vi "Prueba GAP.vi"(11 "Class 2.lvclass":refnum<class "Class 2.lvclass">) -> (3 "Class 2.lvclass 2":refnum<class "Class 2.lvclass">)   [LabVIEW 2019, in "Class 2.lvclass"]
uses:
  Class 2.lvclass
  Class 2.lvclass/Class 2.ctl
panel:
  in  "stop":bool
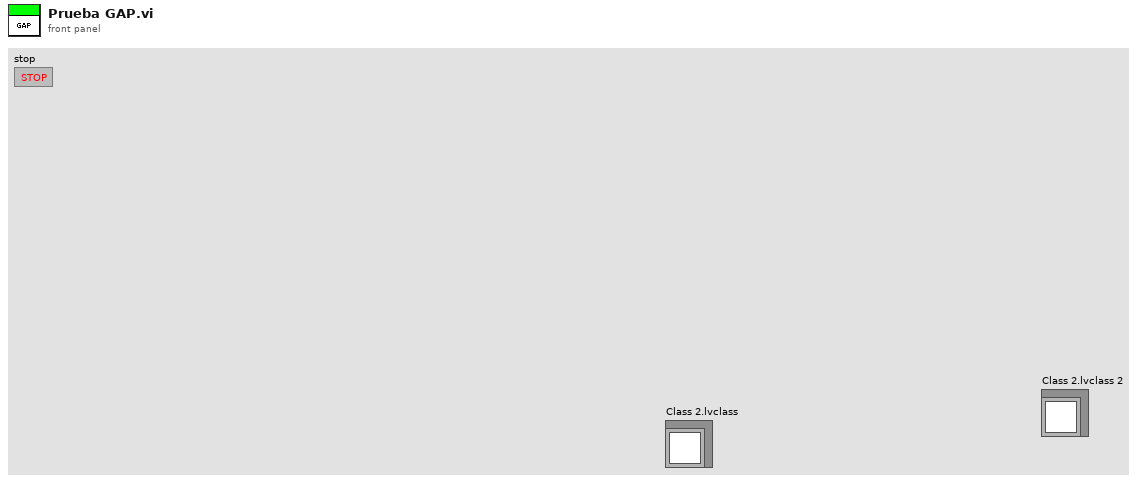
[diagram p1: front panel]
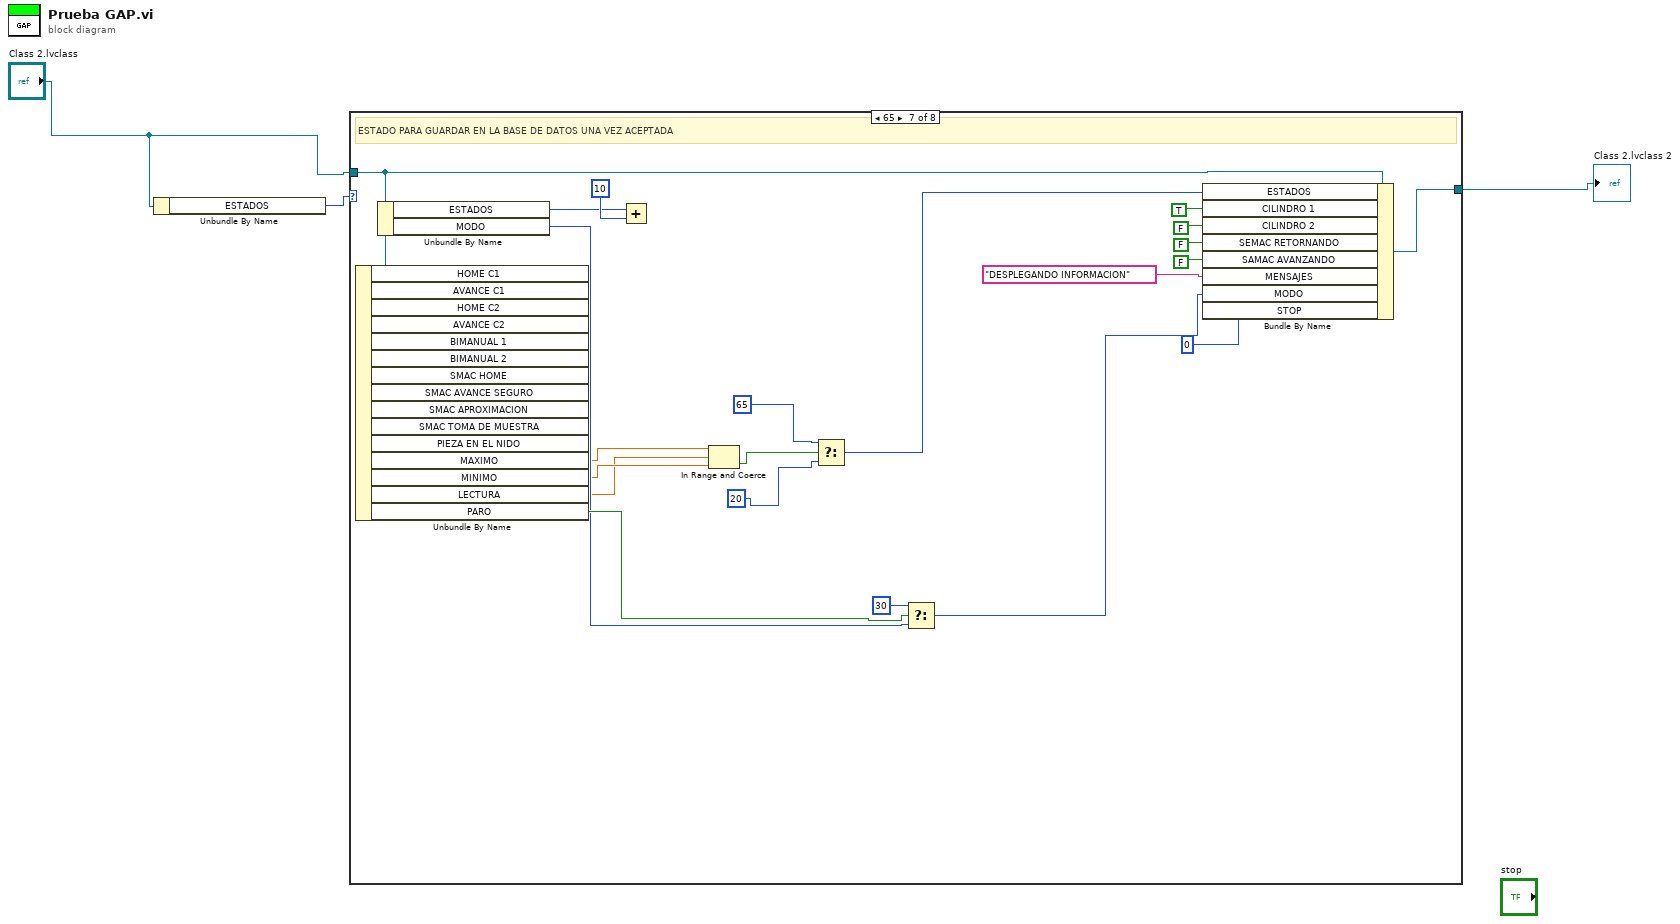
[diagram p0: block diagram]
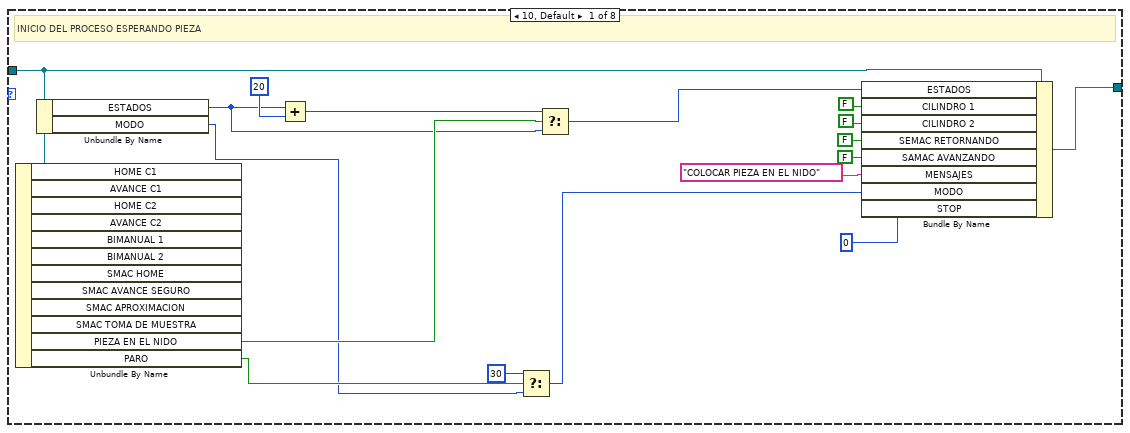
[diagram p2: hidden frame]
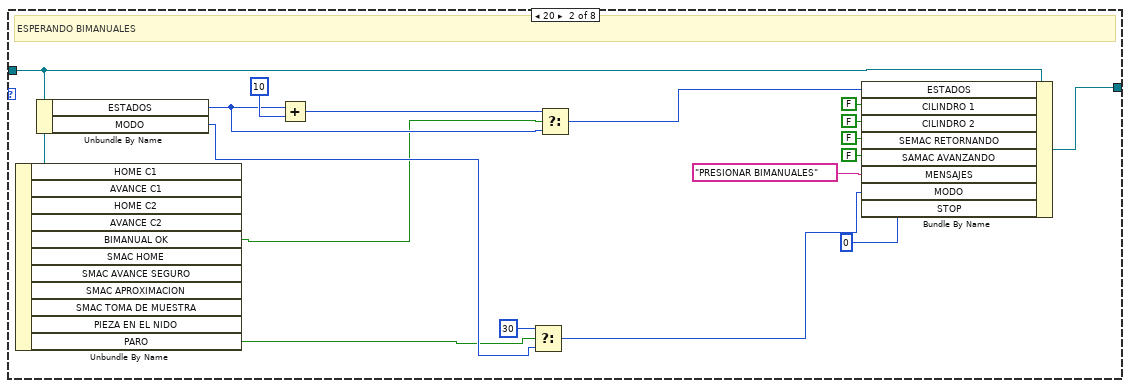
[diagram p3: hidden frame]
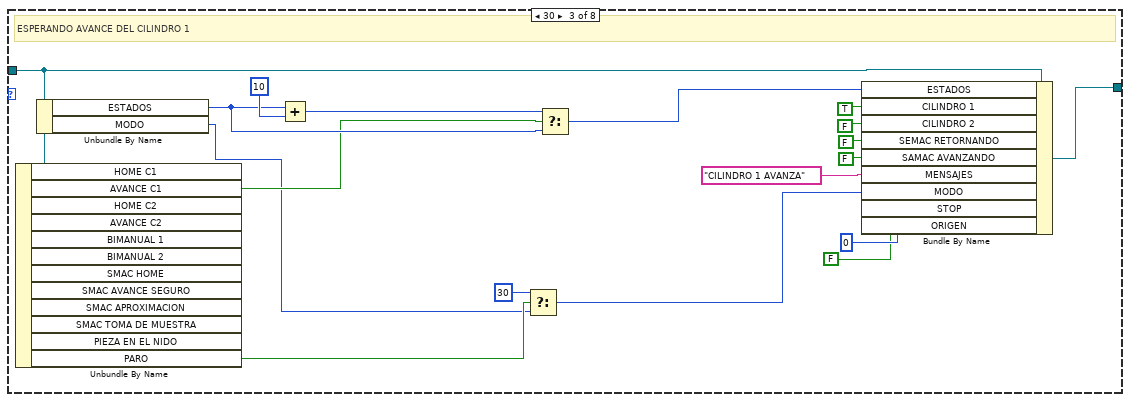
[diagram p4: hidden frame]
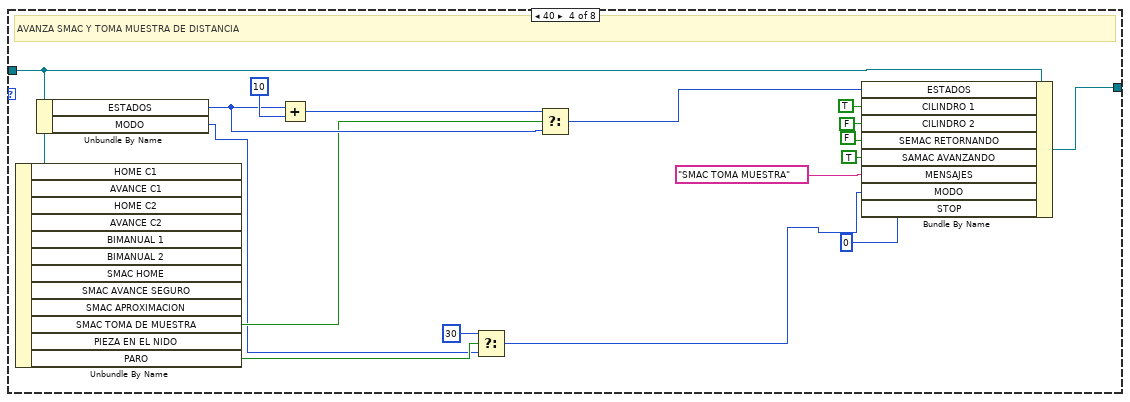
[diagram p5: hidden frame]
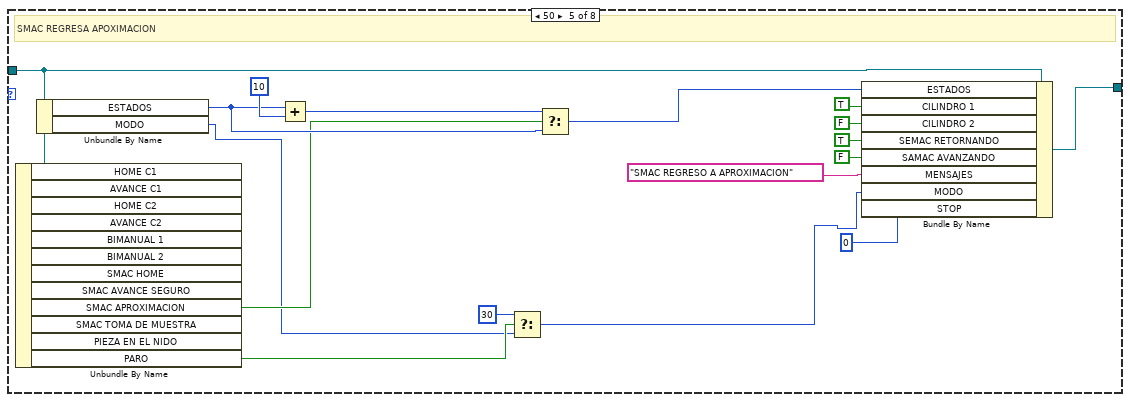
[diagram p6: hidden frame]
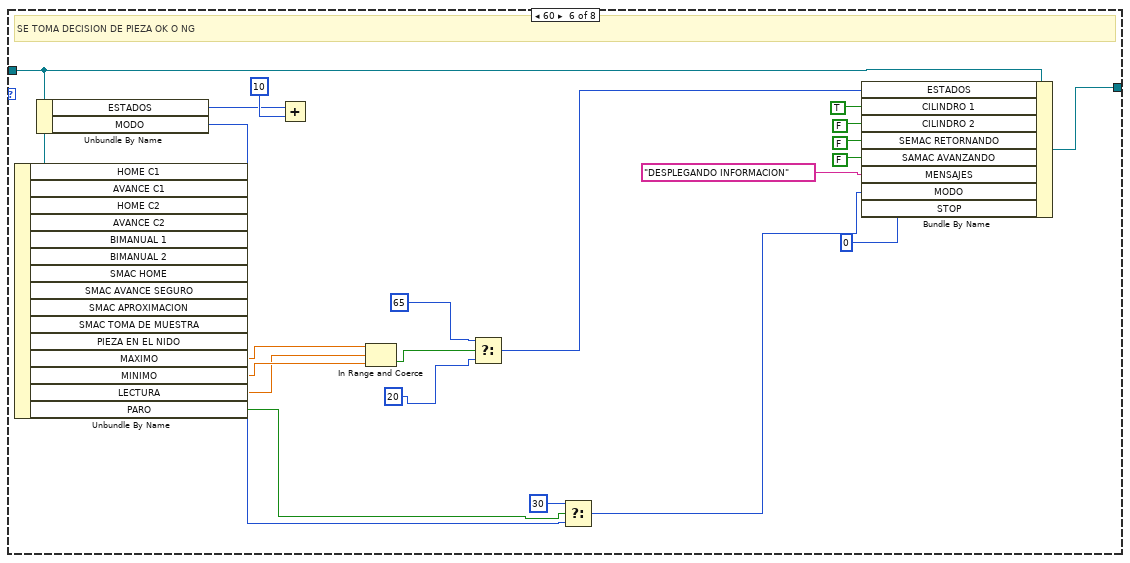
[diagram p7: hidden frame]
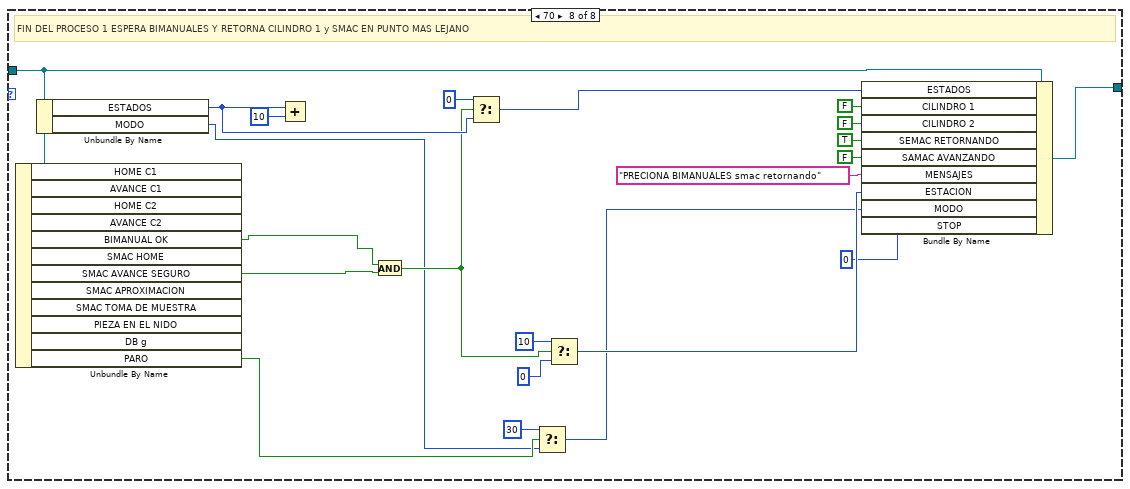
[diagram p8: hidden frame]
diagram:
  n1 = Unbundle By Name("Class 2.lvclass") -> ("ESTADOS"=w3:i16)
  n2 = case shown="65" w3 {
    tunnel: "Class 2.lvclass" -> [w16 w32 w50 w67 w84 w108 w129 w151]
    tunnel: [w20 w37 w55 w72 w89 w110 w131 w153] -> w1
    frame 10, Default {
      # "INICIO DEL PROCESO ESPERANDO PIEZA"
      n3 = Unbundle By Name(w16) -> ("PIEZA EN EL NIDO"=w14:bool, "PARO"=w9:bool)  [unwired: 10 out]
      n4 = Unbundle By Name(w16) -> ("ESTADOS"=w8:i16, "MODO"=w6:i16)
      n5 = Add(x=w8, y=i16 20) -> (x+y=w18:i16)
      n6 = Select(t=i16 30, s=w9, f=w6) -> (s? t:f=w4:i16)
      n7 = Select(t=w18, s=w14, f=w8) -> (s? t:f=w17:i16)
      n8 = Bundle By Name(cluster=w16, "ESTADOS"=w17, "CILINDRO 1"=FALSE ("SALIDAS.CILINDRO 1"), "CILINDRO 2"=FALSE ("SALIDAS.CILINDRO 2"), "SEMAC RETORNANDO"=FALSE ("SALIDAS.SEMAC RETORNANDO"), "SAMAC AVANZANDO"=FALSE ("SALIDAS.SAMAC AVANZANDO"), "MENSAJES"="COLOCAR PIEZA EN EL NIDO" ("SALIDAS.MENSAJES"), "MODO"=w4, "STOP"=i16 0 ("MAQ DE ESTADOS.MODO")) -> (w20:refnum<class "Class 2.lvclass">)
    }
    frame 20 {
      # "ESPERANDO BIMANUALES"
      n9 = Unbundle By Name(w32) -> ("BIMANUAL OK"=w21:bool, "PARO"=w24:bool)  [unwired: 9 out]
      n10 = Unbundle By Name(w32) -> ("ESTADOS"=w34:i16, "MODO"=w25:i16)
      n11 = Add(x=w34, y=i16 10) -> (x+y=w35:i16)
      n12 = Select(t=i16 30, s=w24, f=w25) -> (s? t:f=w23:i16)
      n13 = Select(t=w35, s=w21, f=w34) -> (s? t:f=w33:i16)
      n14 = Bundle By Name(cluster=w32, "ESTADOS"=w33, "CILINDRO 1"=FALSE ("SALIDAS.CILINDRO 1"), "CILINDRO 2"=FALSE ("SALIDAS.CILINDRO 2"), "SEMAC RETORNANDO"=FALSE ("SALIDAS.SEMAC RETORNANDO"), "SAMAC AVANZANDO"=FALSE ("SALIDAS.SAMAC AVANZANDO"), "MENSAJES"="PRESIONAR BIMANUALES" ("SALIDAS.MENSAJES"), "MODO"=w23, "STOP"=i16 0 ("MAQ DE ESTADOS.STOP")) -> (w37:refnum<class "Class 2.lvclass">)
    }
    frame 30 {
      # "ESPERANDO AVANCE DEL CILINDRO 1"
      n15 = Unbundle By Name(w50) -> ("AVANCE C1"=w44:bool, "PARO"=w41:bool)  [unwired: 10 out]
      n16 = Unbundle By Name(w50) -> ("ESTADOS"=w52:i16, "MODO"=w40:i16)
      n17 = Add(x=w52, y=i16 10) -> (x+y=w53:i16)
      n18 = Select(t=i16 30, s=w41, f=w40) -> (s? t:f=w42:i16)
      n19 = Select(t=w53, s=w44, f=w52) -> (s? t:f=w51:i16)
      n20 = Bundle By Name(cluster=w50, "ESTADOS"=w51, "CILINDRO 1"=TRUE ("SALIDAS.CILINDRO 1"), "CILINDRO 2"=FALSE ("SALIDAS.CILINDRO 2"), "SEMAC RETORNANDO"=FALSE ("SALIDAS.SEMAC RETORNANDO"), "SAMAC AVANZANDO"=FALSE ("SALIDAS.SAMAC AVANZANDO"), "MENSAJES"="CILINDRO 1 AVANZA" ("SALIDAS.MENSAJES"), "MODO"=w42, "STOP"=i16 0 ("MAQ DE ESTADOS.STOP"), "ORIGEN"=FALSE ("PROCESO.ORIGEN")) -> (w55:refnum<class "Class 2.lvclass">)
    }
    frame 40 {
      # "AVANZA SMAC Y TOMA MUESTRA DE DISTANCIA"
      n21 = Unbundle By Name(w67) -> ("SMAC TOMA DE MUESTRA"=w61:bool, "PARO"=w59:bool)  [unwired: 10 out]
      n22 = Unbundle By Name(w67) -> ("ESTADOS"=w69:i16, "MODO"=w58:i16)
      n23 = Add(x=w69, y=i16 10) -> (x+y=w70:i16)
      n24 = Select(t=i16 30, s=w59, f=w58) -> (s? t:f=w57:i16)
      n25 = Select(t=w70, s=w61, f=w69) -> (s? t:f=w68:i16)
      n26 = Bundle By Name(cluster=w67, "ESTADOS"=w68, "CILINDRO 1"=TRUE ("SALIDAS.CILINDRO 1"), "CILINDRO 2"=FALSE ("SALIDAS.CILINDRO 2"), "SEMAC RETORNANDO"=FALSE ("SALIDAS.SEMAC RETORNANDO"), "SAMAC AVANZANDO"=TRUE ("SALIDAS.SAMAC AVANZANDO"), "MENSAJES"="SMAC TOMA MUESTRA" ("SALIDAS.MENSAJES"), "MODO"=w57, "STOP"=i16 0 ("MAQ DE ESTADOS.STOP")) -> (w72:refnum<class "Class 2.lvclass">)
    }
    frame 50 {
      # "SMAC REGRESA APOXIMACION"
      n27 = Unbundle By Name(w84) -> ("SMAC APROXIMACION"=w78:bool, "PARO"=w76:bool)  [unwired: 10 out]
      n28 = Unbundle By Name(w84) -> ("ESTADOS"=w86:i16, "MODO"=w75:i16)
      n29 = Add(x=w86, y=i16 10) -> (x+y=w87:i16)
      n30 = Select(t=i16 30, s=w76, f=w75) -> (s? t:f=w74:i16)
      n31 = Select(t=w87, s=w78, f=w86) -> (s? t:f=w85:i16)
      n32 = Bundle By Name(cluster=w84, "ESTADOS"=w85, "CILINDRO 1"=TRUE ("SALIDAS.CILINDRO 1"), "CILINDRO 2"=FALSE ("SALIDAS.CILINDRO 2"), "SEMAC RETORNANDO"=TRUE ("SALIDAS.SEMAC RETORNANDO"), "SAMAC AVANZANDO"=FALSE ("SALIDAS.SAMAC AVANZANDO"), "MENSAJES"="SMAC REGRESO A APROXIMACION" ("SALIDAS.MENSAJES"), "MODO"=w74, "STOP"=i16 0 ("MAQ DE ESTADOS.STOP")) -> (w89:refnum<class "Class 2.lvclass">)
    }
    frame 60 {
      # "SE TOMA DECISION DE PIEZA OK O NG"
      n33 = Unbundle By Name(w108) -> ("MAXIMO"=w96:dbl, "MINIMO"=w95:dbl, "LECTURA"=w94:dbl, "PARO"=w100:bool)  [unwired: 11 out]
      n34 = Unbundle By Name(w108) -> ("ESTADOS"=w102:i16, "MODO"=w99:i16)
      n35 = Add(x=w102, y=i16 10) -> ()  [unwired: 1 out]
      n36 = In Range and Coerce(upper limit=w96, x=w94, lower limit=w95) -> (In Range?=w93:bool)  [unwired: 1 out]
      n37 = Select(t=i16 65 ("y"), s=w93, f=i16 20 ("y")) -> (s? t:f=w90:i16)
      n38 = Select(t=i16 30, s=w100, f=w99) -> (s? t:f=w98:i16)
      n39 = Bundle By Name(cluster=w108, "ESTADOS"=w90, "CILINDRO 1"=TRUE ("SALIDAS.CILINDRO 1"), "CILINDRO 2"=FALSE ("SALIDAS.CILINDRO 2"), "SEMAC RETORNANDO"=FALSE ("SALIDAS.SEMAC RETORNANDO"), "SAMAC AVANZANDO"=FALSE ("SALIDAS.SAMAC AVANZANDO"), "MENSAJES"="DESPLEGANDO INFORMACION" ("SALIDAS.MENSAJES"), "MODO"=w98, "STOP"=i16 0 ("MAQ DE ESTADOS.STOP")) -> (w110:refnum<class "Class 2.lvclass">)
    }
    frame 65 {
      # "ESTADO PARA GUARDAR EN LA BASE DE DATOS UNA VEZ ACEPTADA"
      n40 = Unbundle By Name(w129) -> ("MAXIMO"=w117:dbl, "MINIMO"=w116:dbl, "LECTURA"=w115:dbl, "PARO"=w121:bool)  [unwired: 11 out]
      n41 = Unbundle By Name(w129) -> ("ESTADOS"=w123:i16, "MODO"=w120:i16)
      n42 = Add(x=w123, y=i16 10) -> ()  [unwired: 1 out]
      n43 = In Range and Coerce(upper limit=w117, x=w115, lower limit=w116) -> (In Range?=w114:bool)  [unwired: 1 out]
      n44 = Select(t=i16 65 ("y"), s=w114, f=i16 20 ("y")) -> (s? t:f=w111:i16)
      n45 = Select(t=i16 30, s=w121, f=w120) -> (s? t:f=w119:i16)
      n46 = Bundle By Name(cluster=w129, "ESTADOS"=w111, "CILINDRO 1"=TRUE ("SALIDAS.CILINDRO 1"), "CILINDRO 2"=FALSE ("SALIDAS.CILINDRO 2"), "SEMAC RETORNANDO"=FALSE ("SALIDAS.SEMAC RETORNANDO"), "SAMAC AVANZANDO"=FALSE ("SALIDAS.SAMAC AVANZANDO"), "MENSAJES"="DESPLEGANDO INFORMACION" ("SALIDAS.MENSAJES"), "MODO"=w119, "STOP"=i16 0 ("MAQ DE ESTADOS.STOP")) -> (w131:refnum<class "Class 2.lvclass">)
    }
    frame 70 {
      # "FIN DEL PROCESO 1 ESPERA BIMANUALES Y RETORNA CILINDRO 1 y SMAC EN PUNTO MAS LEJANO"
      n47 = Unbundle By Name(w151) -> ("BIMANUAL OK"=w132:bool, "SMAC AVANCE SEGURO"=w142:bool, "PARO"=w136:bool)  [unwired: 9 out]
      n48 = Unbundle By Name(w151) -> ("ESTADOS"=w144:i16, "MODO"=w135:i16)
      n49 = Add(x=w144, y=i16 10) -> ()  [unwired: 1 out]
      n50 = And(x=w132, y=w142) -> (x .and. y?=w140:bool)
      n51 = Select(t=i16 0, s=w140, f=w144) -> (s? t:f=w145:i16)
      n52 = Select(t=i16 30, s=w136, f=w135) -> (s? t:f=w133:i16)
      n53 = Select(t=i8 10, s=w140, f=i8 0) -> (s? t:f=w138:i8)
      n54 = Bundle By Name(cluster=w151, "ESTADOS"=w145, "CILINDRO 1"=FALSE ("SALIDAS.CILINDRO 1"), "CILINDRO 2"=FALSE ("SALIDAS.CILINDRO 2"), "SEMAC RETORNANDO"=TRUE ("SALIDAS.SEMAC RETORNANDO"), "SAMAC AVANZANDO"=FALSE ("SALIDAS.SAMAC AVANZANDO"), "MENSAJES"="PRECIONA BIMANUALES smac retornando" ("SALIDAS.MENSAJES"), "ESTACION"=w138, "MODO"=w133, "STOP"=i16 0 ("MAQ DE ESTADOS.STOP")) -> (w153:refnum<class "Class 2.lvclass">)
    }
  }
  "Class 2.lvclass 2" <- w1
